vi "Calibration Board.vi"(10 "ARGB Image Source":refnum<data-value>, 11 "UI in":refnum<class "UI.lvclass">) -> ()   [LabVIEW 2020, in "AR Example.lvlib" / "UI.lvclass"]
uses:
  UI.lvclass
  UI.lvclass/UI.ctl
  g_ar_toolkit.image/Image Draw Offset.ctl
  g_ar_toolkit.image/ARGBImageSize.vi
  g_ar_toolkit.image/DrawImageToPictureARGB.vi
  g_ar_toolkit.image/ARGBImageSize.vi/69a1505b-b287-44ed-9ef9-f10ed7b260f4.vi
  g_ar_toolkit.image/DrawImageToPictureARGB.vi/8cd07b1b-062e-4fe4-9e87-2eb3dc89fe0e.vi
  g_ar_toolkit.common/Module Path.vi
  <vilib>/Utility/error.llb/Error Cluster From Error Code.vi
  g_ar_toolkit.image/g_ar_toolkit.image.lvlib
panel:
  out "Calibration Board":picture
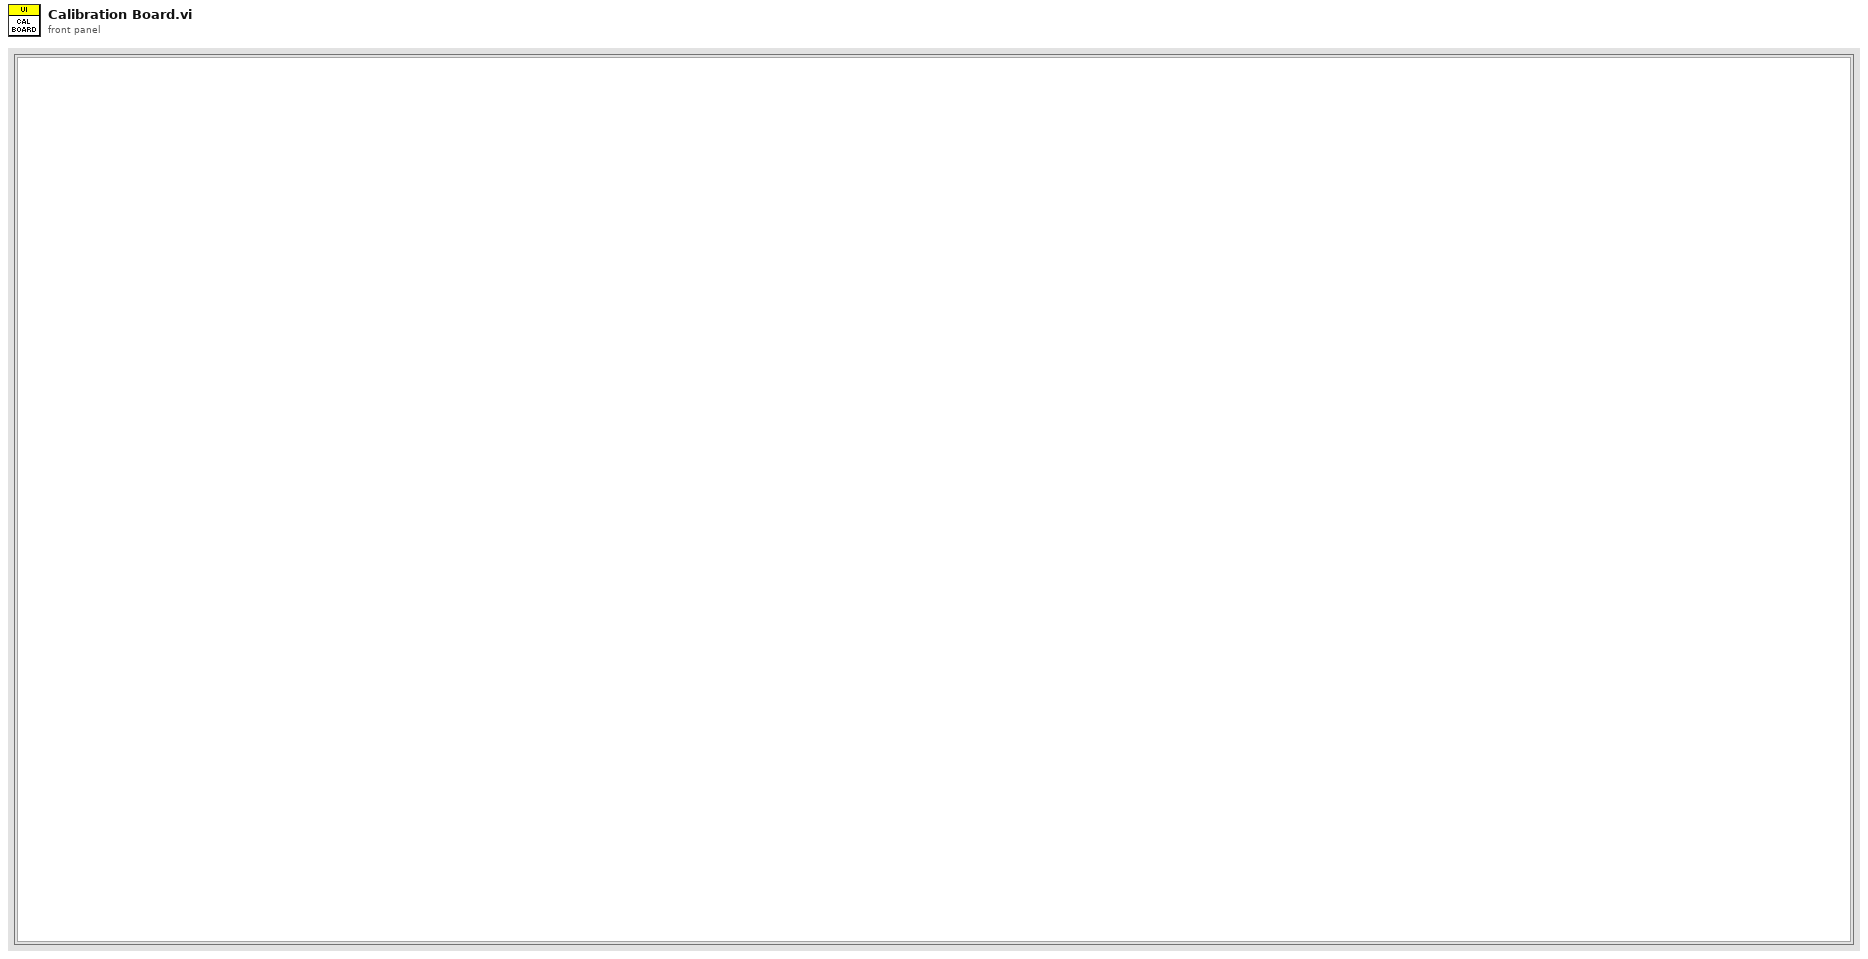
[diagram p1: front panel]
types:
  T1 = typedef "g_ar_toolkit.image.lvlib/Image Draw Offset.ctl" = cluster{"Left":i16, "Top":i16}
  T2 = enum32{"Invalid", "Standard", "Closed", "Hidden", "Minimized", "Maximized"}
  T3 = typedef "g_ar_toolkit.common.lvlib/Image Size (Integer).ctl" = cluster{"Width":u16, "Height":u16}
  T4 = typedef "LVBoundsTypeDef.ctl" = cluster{"Width":u32, "Height":u32}
  T5 = typedef "AR Example.lvlib/UI.lvclass/Calibration Board Events.ctl" = enum16{"Show Panel", "Hide Panel", "Exit"}
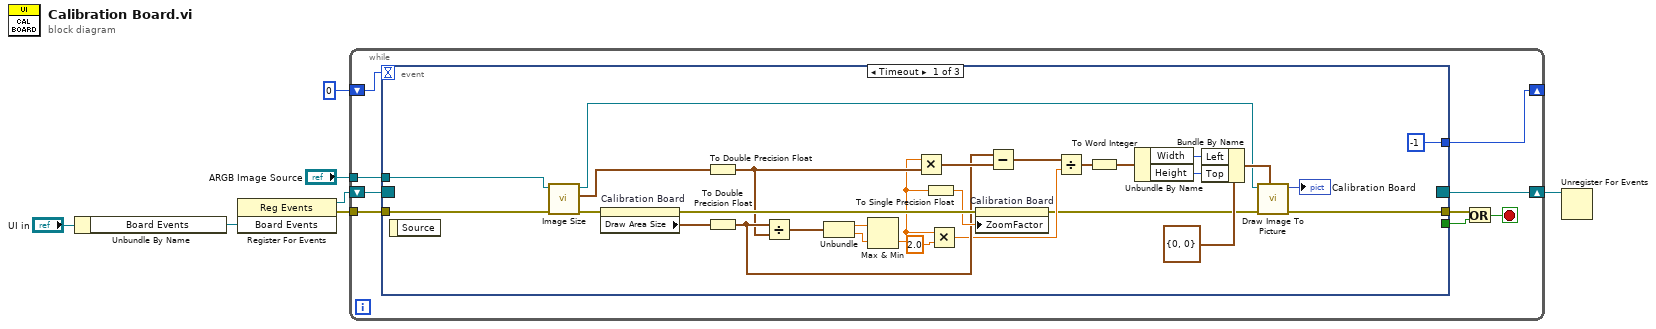
[diagram p0: block diagram]
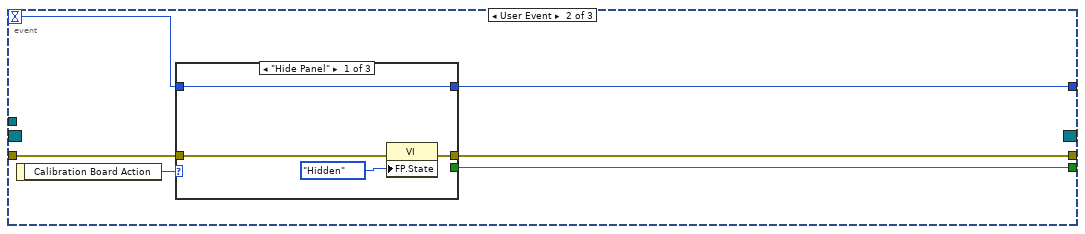
[diagram p2: hidden frame]
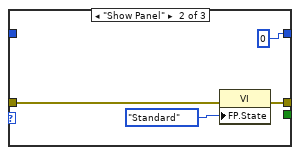
[diagram p3: hidden frame]
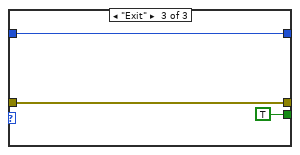
[diagram p4: hidden frame]
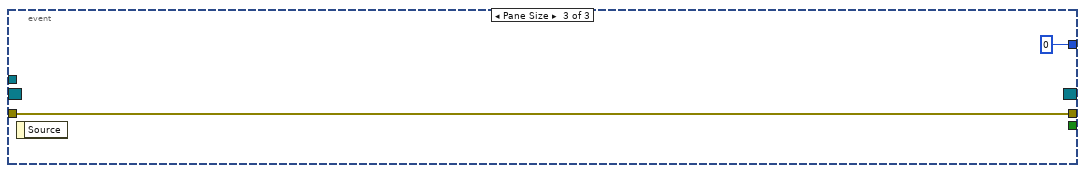
[diagram p5: hidden frame]
diagram:
  n1 = Unbundle By Name("UI in") -> ("Board Events"=w4:refnum<user-event>)
  n2 = register-events(w4) -> (reference out=w2:refnum<event-registration>, error out=w3:errorcluster)  [unwired: 2 in]
  n3 = while {
    shift-right: [w15] -> _
    shift-left: 0 -> [w16]
    tunnel: "ARGB Image Source" -> [w14]
    tunnel: w3 -> [w11]
    shift-right: [w9] -> w1
    shift-left: w2 -> [w10]
    stop <- w12 stop-if-true
    n4 = event shown="[0] Timeout" {
      selector: w10 -> [_ _ _]
      dyn-events: [_ _ _] -> w9
      timeout: w16 -> [_ w45 _]
      tunnel: [-1 w46 0] -> w15
      tunnel: w14 -> [w25 _ _]
      tunnel: [w22 w49 w62] -> w13
      tunnel: w11 -> [w17 w48 w62]
      tunnel: [_ w47 _] -> w8
      event Timeout {
        n5 = event-data() -> ()  [unwired: 1 in, 1 out]
        n6 = call-poly "Image Size.vi"("error in (no error)"=w17, "ARGB Image"=w25) -> ("error out"=w18:errorcluster, "Image Size"=w19:T3, "ARGB Image (duplicate)"=w20:refnum<data-value>)  [unwired: 7 in]
        n7 = property on="Calibration Board" class="Pict"(error in=w18) -> (error out=w40:errorcluster, "Draw Area Size"=w37:T4)  [unwired: 1 in, 1 out]
        n8 = To Double Precision Float(number=w19) -> (double precision float=w34:cluster{"Width":dbl, "Height":dbl})
        n9 = To Double Precision Float(number=w37) -> (double precision float=w35:cluster{"Width":dbl, "Height":dbl})
        n10 = Divide(x=w35, y=w34) -> (x/y=w43:cluster{"Width":dbl, "Height":dbl})
        n11 = Unbundle(w43) -> ("Width"=w41:dbl, "Height"=w42:dbl)
        n12 = Max & Min(x=w41, y=w42) -> (min(x,y)=w26:dbl)  [unwired: 1 out]
        n13 = Multiply(x=w26, y=w34) -> (x*y=w38:cluster{"Width":dbl, "Height":dbl})
        n14 = To Single Precision Float(number=w26) -> (single precision float=w39:sgl)
        n15 = Multiply(x=w26, y=2.0) -> (x*y=w27:dbl)
        n16 = property on="Calibration Board" class="Pict"(error in=w40, "ZoomFactor"=w39) -> (error out=w24:errorcluster)  [unwired: 1 in, 1 out]
        n17 = Subtract(x=w35, y=w38) -> (x-y=w36:cluster{"Width":dbl, "Height":dbl})
        n18 = Divide(x=w36, y=w27) -> (x/y=w32:cluster{"Width":dbl, "Height":dbl})
        n19 = To Word Integer(number=w32) -> (16bit integer=w30:cluster{"Width":i16, "Height":i16})
        n20 = Unbundle By Name(w30) -> ("Width"=w29:i16, "Height"=w28:i16)
        n21 = Bundle By Name(cluster=T1 {"Left"=0, "Top"=0} ("Image Draw Offset"), "Left"=w29, "Top"=w28) -> (w23:T1)
        n22 = call-poly "Draw Image To Picture.vi"("Image Draw Offset (Default 0,0)"=w23, "error in (no error)"=w24, "ARGB Image Source"=w20) -> ("error out"=w22:errorcluster, "Picture"=→"Calibration Board":picture)  [unwired: 7 in]
      }
      event User Event {
        n23 = event-data() -> ("Calibration Board Action"=w50:T5)  [unwired: 1 in]
        n24 = case shown="\"Hide Panel\"" w50 {
          tunnel: [w53 w57 w61] -> w49
          tunnel: w48 -> [w52 w56 w61]
          tunnel: [_ _ TRUE] -> w47
          tunnel: [w51 0 w59] -> w46
          tunnel: w45 -> [w51 _ w59]
          frame "Hide Panel" {
            n25 = property class="VI"(error in=w52, "FP.State"=T2."Hidden" ("Front Panel Window:State")) -> (error out=w53:errorcluster)  [unwired: 1 in, 1 out]
          }
          frame "Show Panel" {
            n26 = property class="VI"(error in=w56, "FP.State"=T2."Standard" ("Front Panel Window:State")) -> (error out=w57:errorcluster)  [unwired: 1 in, 1 out]
          }
          frame "Exit" {
          }
        }
      }
      event Pane Size {
        n27 = event-data() -> ()  [unwired: 1 in, 1 out]
      }
    }
    n28 = Or(x=w13, y=w8) -> (x .or. y?=w12:bool)
  }
  n29 = Unregister For Events(event registration refnum=w1) -> ()  [unwired: 1 in, 1 out]
